vi "calculate_r_squared.vi"(8 "Error In":errorcluster, 10 "Expected":dbl[](array[numeric]), 11 "Fits":dbl[](array[numeric])) -> (0 "Error Out":errorcluster, 3 "R2":dbl)   [LabVIEW 2019]
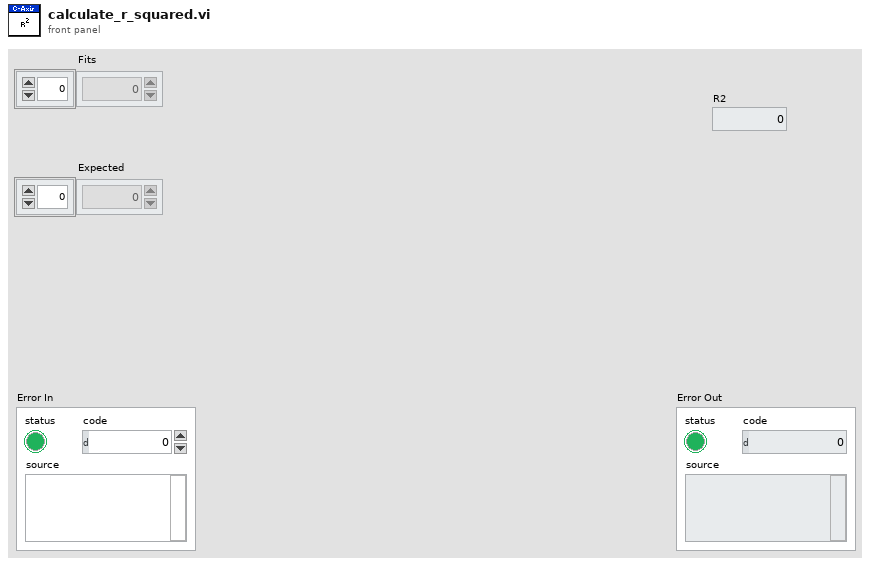
[diagram p1: front panel]
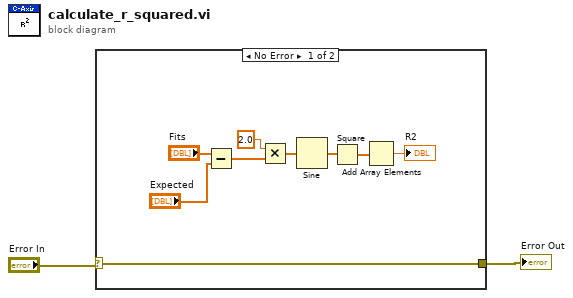
[diagram p0: block diagram]
diagram:
  n1 = case shown="No Error" "Error In" {
    selector: "Error In" -> [w3 w12]
    tunnel: [w3 w12] -> w1
    frame No Error {
      n2 = Subtract(x="Fits", y="Expected") -> (x-y=w11:dbl[])
      n3 = Multiply(x=2.0, y=w11) -> (x*y=w9:dbl[])
      n4 = Sine(x=w9) -> (sin(x)=w8:dbl[])
      n5 = Square(x=w8) -> (x^2=w7:dbl[])
      n6 = Add Array Elements(numeric array=w7) -> (sum=→"R2":dbl)
    }
    frame Error {
    }
  }
  "Error Out" <- w1
